vi "WSVCAP SHL Host LL I2C Build and Parse Write Message.vi"(0 "C1 Write Data In [DUT Ordered]":u8[][](array[numeric]) format="%.0x", 1 "Message In":string, 2 "UUT Set (0/1) In":u8=20 format="%.0x", 5 "C2 Write Data [DUT Ordered]":u8[][](array[numeric]) format="%.0x", 7 "C3Write Data [DUT Ordered]":u8[][](array[numeric]) format="%.0x", 9 "Socket Mask [U64] In":u64=1 format="%016x", 11 "error in":errorcluster, 12 "Sub Address In":u8=20 format="%.0x") -> (3 "Message Out":string, 4 "C1 Write Data Out [DUT Ordered]":u8[][](array[numeric]) format="%.0x", 6 "C2 Write Data Out [DUT Ordered]":u8[][](array[numeric]) format="%.0x", 8 "C3 Write Data Out [DUT Ordered]":u8[][](array[numeric]) format="%.0x", 10 "Socket Mask [U64] Out":u64=1 format="%08x", 13 "UUT Set (0/1) Out":u8=20 format="%.0x", 14 "Sub Address Out":u8=20 format="%.0x", 15 "error out":errorcluster)   [LabVIEW 2012]
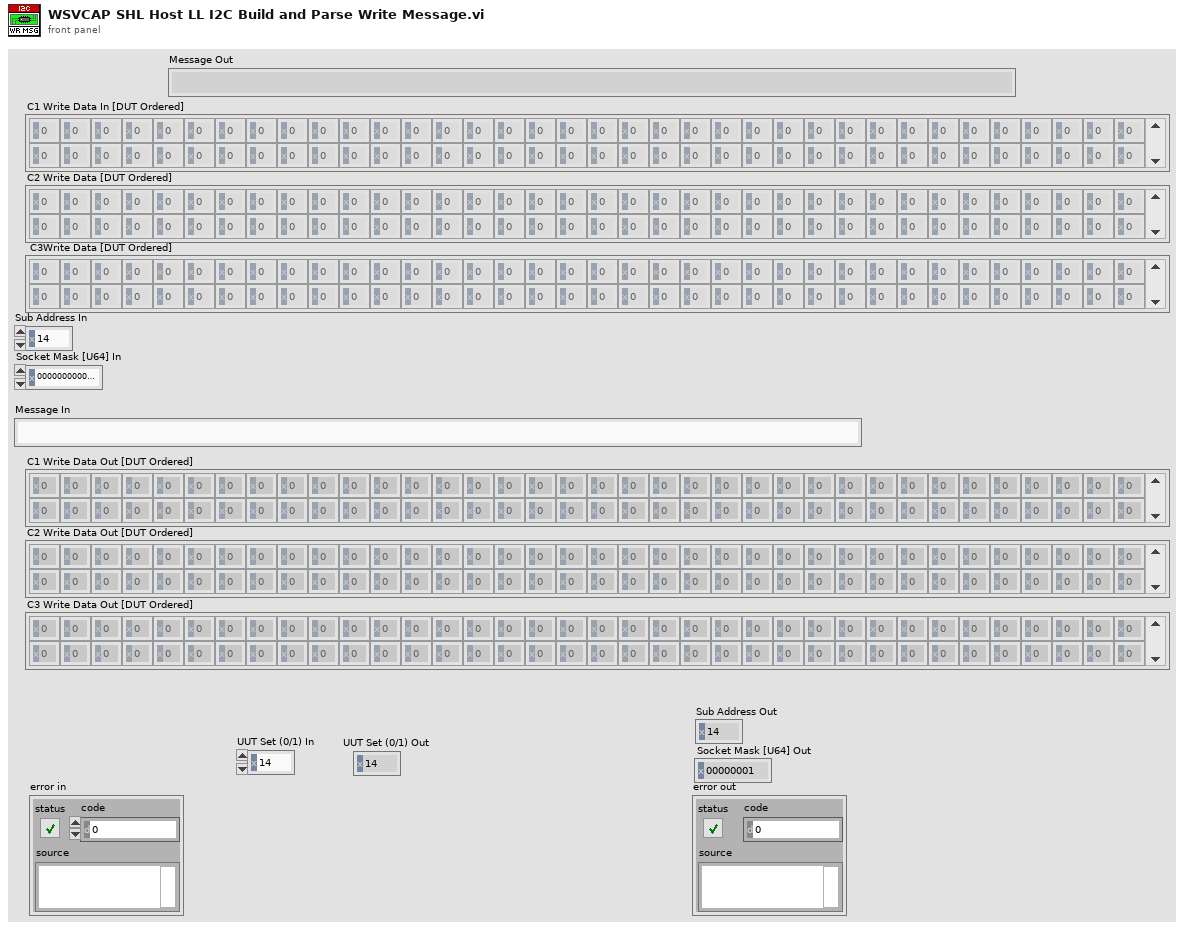
[diagram p1: front panel]
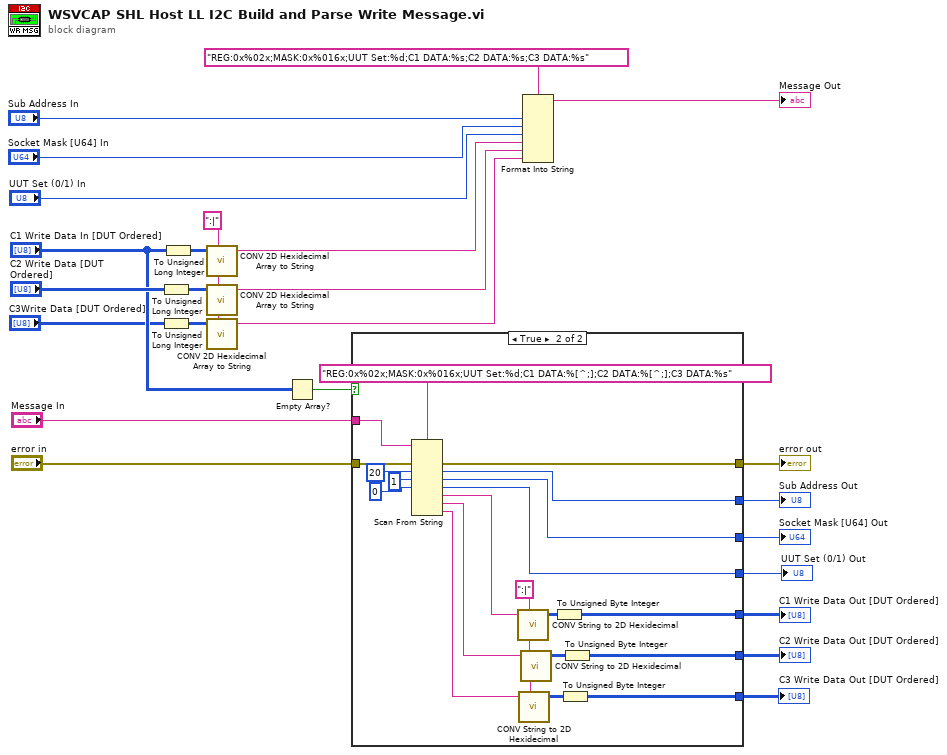
[diagram p0: block diagram]
diagram:
  w5 = ":|" ("Delimiters (,;)")
  n1 = To Unsigned Long Integer(number="C2 Write Data [DUT Ordered]") -> (unsigned 32bit integer=w7:u32[][])
  n2 = To Unsigned Long Integer(number="C3Write Data [DUT Ordered]") -> (unsigned 32bit integer=w8:u32[][])
  n3 = To Unsigned Long Integer(number="C1 Write Data In [DUT Ordered]") -> (unsigned 32bit integer=w25:u32[][])
  n4 = call "CONV 2D Hexidecimal Array to String.vi"("2-D Hexidecimal"=w25, "Delimiters (,;)"=w5) -> ("String"=w21:string)  [unwired: 7 in]
  n5 = call "CONV 2D Hexidecimal Array to String.vi"("2-D Hexidecimal"=w7, "Delimiters (,;)"=w5) -> ("String"=w20:string)  [unwired: 7 in]
  n6 = call "CONV 2D Hexidecimal Array to String.vi"("2-D Hexidecimal"=w8, "Delimiters (,;)"=w5) -> ("String"=w4:string)  [unwired: 7 in]
  n7 = Empty Array?(array="C1 Write Data In [DUT Ordered]") -> (empty?=w9:bool)
  n8 = case shown="True" w9 {
    tunnel: [_ w44] -> w18
    tunnel: [_ w43] -> w17
    tunnel: [_ w41] -> w16
    tunnel: [_ w40] -> w15
    tunnel: "error in" -> [w26 w37]
    tunnel: [w26 w36] -> w12
    tunnel: "Message In" -> [_ w35]
    tunnel: [_ w29] -> w3
    tunnel: [_ w27] -> w1
    frame False {
    }
    frame True {
      w30 = ":|" ("Delimiters (,;)")
      n9 = Scan From String(format string="REG:0x%02x;MASK:0x%016x;UUT Set:%d;C1 DATA:%[^;];C2 DATA:%[^;];C3 DATA:%s", input string=w35, error in=w37, default 1=u8 20 ("Sub Address Out"), default 2=u64 1 ("Socket Mask [U32] Out"), default 3=u8 0 ("Sub Address Out")) -> (error out=w36:errorcluster, output 1=w41:u8, output 2=w40:u64, output 3=w27:u8, output 4=w39:string, output 5=w38:string, output 6=w31:string)  [unwired: 4 in, 2 out]
      n10 = call "CONV String to 2D Hexidecimal.vi"("String"=w39, "Delimiters (,;)"=w30) -> ("2-D Hexidecimal"=w46:u32[][])  [unwired: 7 in]
      n11 = call "CONV String to 2D Hexidecimal.vi"("String"=w31, "Delimiters (,;)"=w30) -> ("2-D Hexidecimal"=w32:u32[][])  [unwired: 7 in]
      n12 = call "CONV String to 2D Hexidecimal.vi"("String"=w38, "Delimiters (,;)"=w30) -> ("2-D Hexidecimal"=w45:u32[][])  [unwired: 7 in]
      n13 = To Unsigned Byte Integer(number=w46) -> (unsigned 8bit integer=w44:u8[][])
      n14 = To Unsigned Byte Integer(number=w32) -> (unsigned 8bit integer=w29:u8[][])
      n15 = To Unsigned Byte Integer(number=w45) -> (unsigned 8bit integer=w43:u8[][])
    }
  }
  "C1 Write Data Out [DUT Ordered]" <- w18
  "C2 Write Data Out [DUT Ordered]" <- w17
  "Sub Address Out" <- w16
  "Socket Mask [U64] Out" <- w15
  "error out" <- w12
  "C3 Write Data Out [DUT Ordered]" <- w3
  "UUT Set (0/1) Out" <- w1
  n16 = Format Into String(format string="REG:0x%02x;MASK:0x%016x;UUT Set:%d;C1 DATA:%s;C2 DATA:%s;C3 DATA:%s", "Sub Address In", "Socket Mask [U64] In", "UUT Set (0/1) In", w21, w20, w4) -> (resulting string=→"Message Out":string)  [unwired: 2 in, 1 out]
